vi "Main On Compile Action VI.vi"(8 "error in (no error)":errorcluster, 11 "Device Item Ref in":T1 format="%.0x") -> (0 "error out":errorcluster)   [LabVIEW 2011, in "Engine Sim System Explorer.lvlib"]
uses:
  Engine Sim System Explorer.lvlib
  <vilib>/NI Veristand/Custom Device API/Custom Device Item Ref.ctl
  <vilib>/NI Veristand/Custom Device API/Custom Device Channel Type.ctl
  Shared/Channel Descriptors.ctl
  Shared/FPGA Write Descriptor.ctl
  Shared/InputChannelTypes.ctl
  <vilib>/rvi/DataTransferAndStorage/Container/Common/niFpgaDataTypeControl.ctl
  Shared/FPGA Read Descriptor.ctl
  Shared/OutputChannelTypes.ctl
  Shared/Status Chan Descriptor.ctl
  Shared/EngineSimConfig.ctl
  Shared/NTeethConfig.ctl
  Shared/FullyCustomConfig.ctl
  Shared/FullyCustomProfileConfig.ctl
  Shared/FullyCustomCommMode.ctl
  Shared/DataReplayLoopConfig.ctl
  Shared/DataReplayConfig.ctl
  Shared/DataReplayVoltageConfig.ctl
  Shared/Engine Simulation Global.vi
  <vilib>/NI Veristand/Custom Device API/Set Item Property (Variant).vi
  <vilib>/NI Veristand/Custom Device API/Get Item Property (Boolean).vi
  <vilib>/NI Veristand/Custom Device API/Get Item Property (Dependent Node Pointer).vi
  Engine Simulation Shared.lvlib
  <vilib>/NI Veristand/Custom Device API/Custom Device API.lvlib
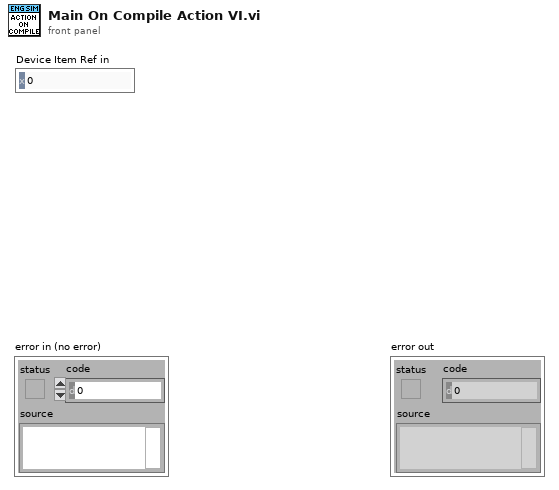
[diagram p1: front panel]
types:
  T1 = typedef "Custom Device API.lvlib/Custom Device Item Ref.ctl" = u64
  T2 = typedef "Custom Device API.lvlib/Custom Device Channel Type.ctl" = enum16{"Input", "Output"}
  T3 = typedef "Engine Simulation Shared.lvlib/Channel Descriptors.ctl" = cluster{"Write Descriptors":T4[], "Read Descriptors":T7[], "Status Descriptor":T9}
  T4 = typedef "Engine Simulation Shared.lvlib/FPGA Write Descriptor.ctl" = cluster{"Register Type":T5, "Address":u32, "FIFO Idx":i32, "OldVal":dbl, "Reg Name":string, "Data Type":T6}
  T5 = typedef "Engine Simulation Shared.lvlib/InputChannelTypes.ctl" = enum16{"Engine Speed", "Offset"}
  T6 = typedef "niFpgaDataTypeControl.ctl" = enum32{"Boolean", "I8", "I16", "I32", "I64", "U8", "U16", "U32", "U64", "FXP", "CustomControl"}
  T7 = typedef "Engine Simulation Shared.lvlib/FPGA Read Descriptor.ctl" = cluster{"Register Type":T8, "Register Address":u32, "FIFO Idx":i32, "DurationMultiplier":dbl, "Reg Name":string, "Data Type":T6}
  T8 = typedef "Engine Simulation Shared.lvlib/OutputChannelTypes.ctl" = enum16{"Cycle Angle", "Crank Angle", "Time Duration", "Angle Duration", "Start Angle", "End Angle"}
  T9 = typedef "Engine Simulation Shared.lvlib/Status Chan Descriptor.ctl" = cluster{"ErrorIDx":i32, "CountIDx":i32, "DurationIDx":i32}
  T10 = typedef "Engine Simulation Shared.lvlib/EngineSimConfig.ctl" = cluster{"NTeeth Configs":T11[], "FullyCustom Configs":T12[], "DataReplayLoops":T15[], "APU.IncrementRate":u64, "DataReplayVoltages":T17[], "Channel Descriptors":T3, "Inputs":i32, "Outputs":i32}
  T11 = typedef "Engine Simulation Shared.lvlib/NTeethConfig.ctl" = cluster{"Base Path":string, "Degrees High Pulse":u64, "Degrees Low Pulse":u64, "TopDeadCenter High?":bool, "Num Teeth Miss":u8, "Missing Teeth Offset":u64, "TDC Offset":u64}
  T12 = typedef "Engine Simulation Shared.lvlib/FullyCustomConfig.ctl" = cluster{"Base Path":string, "Num Profiles":u8, "Num Angles":u8, "Profile Configs":T13[], "Angles FIFO":u64[], "Comm Mode":T14}
  T13 = typedef "Engine Simulation Shared.lvlib/FullyCustomProfileConfig.ctl" = cluster{"Base Path":string, "First Rising?":bool}
  T14 = typedef "Engine Simulation Shared.lvlib/FullyCustomCommMode.ctl" = enum16{"DMA FIFO", "FP Data Transfer"}
  T15 = typedef "Engine Simulation Shared.lvlib/DataReplayLoopConfig.ctl" = cluster{"UpdateRatePath":string, "Loop Tics":u32, "Profile Configs":T16[]}
  T16 = typedef "Engine Simulation Shared.lvlib/DataReplayConfig.ctl" = cluster{"RPMThreshPath":string, "Data":i16[], "VScaleM":u32, "AngleToAdds":u32, "RPMThresh":u64, "NumStr":string, "Number":i8, "AngleToAddsPath":string, "VScaleMPath":string, "VScaleB":i32, "VScaleBPath":string, "CycleAngle?":bool, "CycleAnglePath":string, "ReverseNegate?":bool, "ReverseNegatePath":string}
  T17 = typedef "Engine Simulation Shared.lvlib/DataReplayVoltageConfig.ctl" = cluster{"VScaleMPath":string, "VScaleBPath":string, "DefaultVScaleM":u32, "DefaultVScaleB":i32, "EnableFIFOIdx":i32, "MFIFOIdx":i32, "BFIFOIdx":i32, "Reset":bool, "MAddress":u32, "BAddress":u32}
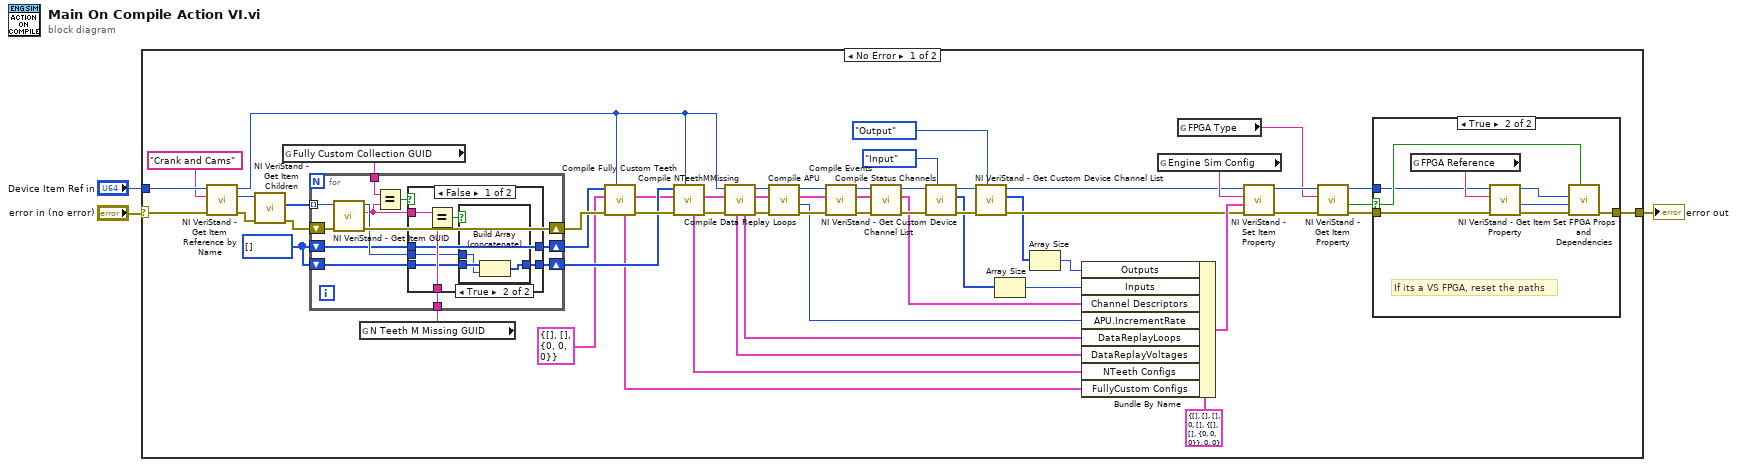
[diagram p0: block diagram]
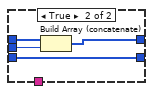
[diagram p4: hidden frame]
diagram:
  n1 = case shown="No Error" "error in (no error)" {
    selector: "error in (no error)" -> [w57 w96]
    tunnel: [w35 w96] -> w2
    tunnel: "Device Item Ref in" -> [w59 _]
    frame No Error {
      w51 = T1[] []
      n2 = call <vilib>:"NI VeriStand - Get Item Reference by Name.vi"("error in (no error)"=w57, "Item Name"="Crank and Cams", "Parent Ref in"=w59) -> ("error out"=w55:errorcluster, "Item Ref"=w56:T1, "Parent Ref out"=w4:T1)  [unwired: 5 in, 1 out]
      n3 = call <vilib>:"NI VeriStand - Get Item Children.vi"("error in (no error)"=w55, "Item Ref in"=w56) -> ("error out"=w53:errorcluster, "Child Refs"=w54:T1[])  [unwired: 6 in, 2 out]
      n4 = global read "Engine Simulation Global.vi" "Fully Custom Collection GUID"() -> (w52:string)
      n5 = global read "Engine Simulation Global.vi" "N Teeth M Missing GUID"() -> (w50:string)
      n6 = for {
        tunnel: w54 -> [w80] mode=indexing
        shift-right: [w78] -> w49
        shift-left: w53 -> [w79]
        tunnel: w52 -> [w77]
        shift-right: [w74] -> w48
        shift-left: w51 -> [w73]
        shift-right: [w69] -> w46
        shift-left: w51 -> [w70]
        tunnel: w50 -> [w71]
        n7 = call <vilib>:"NI VeriStand - Get Item GUID.vi"("error in (no error)"=w79, "Item Ref in"=w80) -> ("error out"=w78:errorcluster, "GUID"=w72:string, "Item Ref out"=w75:T1)  [unwired: 7 out]
        n8 = Equal?(x=w77, y=w72) -> (x = y?=w76:bool)
        n9 = case shown="False" w76 {
          tunnel: w75 -> [w82 w95]
          tunnel: [w85 w94] -> w74
          tunnel: w73 -> [w85 w93]
          tunnel: w72 -> [w87 _]
          tunnel: w71 -> [w86 _]
          tunnel: w70 -> [w83 w92]
          tunnel: [w81 w92] -> w69
          frame False {
            n10 = Equal?(x=w87, y=w86) -> (x = y?=w84:bool)
            n11 = case shown="True" w84 {
              tunnel: w83 -> [w88 w91]
              tunnel: w82 -> [_ w90]
              tunnel: [w88 w89] -> w81
              frame False {
              }
              frame True {
                n12 = Build Array (concatenate)(w91, w90) -> (w89:T1[])
              }
            }
          }
          frame True {
            n13 = Build Array (concatenate)(w93, w95) -> (w94:T1[])
          }
        }
      }
      n14 = call "Compile Fully Custom Teeth.vi"("Custom Device Ref"=w4, "error in (no error)"=w49, "Channel Descriptors in"=T3 {"Write Descriptors"=[], "Read Descriptors"=[], "Status Descriptor"={"ErrorIDx"=0, "CountIDx"=0, "DurationIDx"=0}} ("Channel Descriptors"), "Fully custom teeth refs"=w48) -> ("error out"=w47:errorcluster, "Channel Descriptors out"=w24:T3, "Fully Custom Teeth"=w29:T12[])  [unwired: 5 in]
      n15 = call "Compile NTeethMMissing.vi"("Custom Device Ref"=w4, "error in (no error)"=w47, "Channel Descriptors in"=w24, "N Teeth M Missing refs"=w46) -> ("error out"=w44:errorcluster, "Channel Descriptors out"=w23:T3, "N Teeth M Missing"=w28:T11[])  [unwired: 5 in]
      n16 = call "Compile Data Replay Loops.vi"("error in (no error)"=w44, "Channel Descriptors in"=w23, "Custom Device Ref"=w4) -> ("error out"=w32:errorcluster, "Channel Descriptors out"=w6:T3, "Custom Device Ref dup"=w33:T1, "DataReplayLoops"=w26:T15[], "DataReplayVoltages"=w27:T17[])  [unwired: 4 in]
      n17 = call "Compile APU.vi"("error in (no error)"=w32, "Channel Descriptors in"=w6, "Custom Device Ref in"=w33) -> ("error out"=w34:errorcluster, "IncrementRate"=w7:i64, "Channel Descriptors out"=w5:T3, "Custom Device Ref out"=w30:T1)  [unwired: 5 in]
      n18 = call "Compile Events.vi"("error in (no error)"=w34, "Channel Descriptors in"=w5, "Custom Device Ref"=w30) -> ("error out"=w31:errorcluster, "Channel Descriptors out"=w20:T3, "Custom Device Ref dup"=w21:T1)  [unwired: 6 in]
      n19 = call "Compile Status Channels.vi"("error in (no error)"=w31, "Channel Descriptors in"=w20, "Custom Device Ref"=w21) -> ("error out"=w22:errorcluster, "Channel Descriptors out"=w19:T3, "Custom Device Ref dup"=w17:T1)  [unwired: 6 in]
      n20 = call <vilib>:"NI VeriStand - Get Custom Device Channel List.vi"("Channel Type"=Custom_Device_Channel_Type."Input", "error in (no error)"=w22, "Device Ref in"=w17) -> ("error out"=w18:errorcluster, "Specified Channel Ref List"=w11:T1[], "Device Ref out"=w15:T1)  [unwired: 6 in]
      n21 = call <vilib>:"NI VeriStand - Get Custom Device Channel List.vi"("Channel Type"=Custom_Device_Channel_Type."Output", "error in (no error)"=w18, "Device Ref in"=w15) -> ("error out"=w16:errorcluster, "Specified Channel Ref List"=w8:T1[], "Device Ref out"=w14:T1)  [unwired: 6 in]
      n22 = Array Size(array=w11) -> (size(s)=w10:i32)
      n23 = Array Size(array=w8) -> (size(s)=w9:i32)
      n24 = Bundle By Name(cluster=T10 {"NTeeth Configs"=[], "FullyCustom Configs"=[], "DataReplayLoops"=[], "APU.IncrementRate"=0, "DataReplayVoltages"=[], "Channel Descriptors"={"Write Descriptors"=[], "Read Descriptors"=[], "Status Descriptor"={"ErrorIDx"=0, "CountIDx"=0, "DurationIDx"=0}}, "Inputs"=0, "Outputs"=0} ("Engine Sim Config"), "Outputs"=w9, "Inputs"=w10, "Channel Descriptors"=w19, "APU.IncrementRate"=w7, "DataReplayLoops"=w26, "DataReplayVoltages"=w27, "NTeeth Configs"=w28, "FullyCustom Configs"=w29) -> (w43:T10)
      n25 = global read "Engine Simulation Global.vi" "Engine Sim Config"() -> (w42:string)
      n26 = global read "Engine Simulation Global.vi" "FPGA Type"() -> (w39:string)
      n27 = call-poly <vilib>:"NI VeriStand - Set Item Property.vi"("error in (no error)"=w16, "Value"=w43, "Property Name"=w42, "Item Ref in"=w14) -> ("error out"=w41:errorcluster, "Item Ref out"=w40:T1)  [unwired: 5 in, 1 out]
      n28 = call-poly <vilib>:"NI VeriStand - Get Item Property.vi"("error in (no error)"=w41, "Property Name"=w39, "Item Ref in"=w40) -> ("error out"=w37:errorcluster, "Value"=w38:bool, "Item Ref out"=w36:T1)  [unwired: 5 in, 1 out]
      n29 = case shown="True" w38 {
        selector: w38 -> [_ w66]
        tunnel: w37 -> [w60 w63]
        tunnel: w36 -> [_ w62]
        tunnel: [w60 w61] -> w35
        frame False {
        }
        frame True {
          # "If its a VS FPGA, reset the paths"
          n30 = global read "Engine Simulation Global.vi" "FPGA Reference"() -> (w68:string)
          n31 = call-poly <vilib>:"NI VeriStand - Get Item Property.vi"("error in (no error)"=w63, "Property Name"=w68, "Item Ref in"=w62) -> ("error out"=w67:errorcluster, "Dependent Node Ref"=w64:T1, "Item Ref out"=w65:T1)  [unwired: 5 in, 1 out]
          n32 = call "Set FPGA Props and Dependencies.vi"("VS FPGA?"=w66, "error in (no error)"=w67, "FPGA Ref"=w64, "CD Ref in"=w65) -> ("error out"=w61:errorcluster)  [unwired: 6 in, 1 out]
        }
      }
    }
    frame Error {
    }
  }
  "error out" <- w2
